vi "Set Serial Settings.vi"(8 "error in (no error)":errorcluster, 11 "LightBox in":refnum<class "LightBox.lvclass">=refnum) -> (0 "error out":errorcluster, 3 "LightBox out":refnum<class "LightBox.lvclass">)   [LabVIEW 2016, in "LightBox.lvclass"]
uses:
  LightBox.lvclass
  Quartz/Quartz.lvclass
  Desktop/platinum-modbus-driver/omega_engineering-platinum-modbus-driver-671bd10261c3/Labview Source Code/Platinum Serial Modbus/Platinum_MB_serMode.ctl
  Desktop/platinum-modbus-driver/omega_engineering-platinum-modbus-driver-671bd10261c3/Labview Source Code/Platinum Serial Modbus/Platinum_MB_serFlowControl.ctl
  Desktop/platinum-modbus-driver/omega_engineering-platinum-modbus-driver-671bd10261c3/Labview Source Code/Platinum Serial Modbus/Platinum_MB_SerHandle.ctl
  Desktop/platinum-modbus-driver/omega_engineering-platinum-modbus-driver-671bd10261c3/Labview Source Code/Platinum Serial Modbus/Platinum_MB_serParity.ctl
  LightBox.lvclass/LightBox.ctl
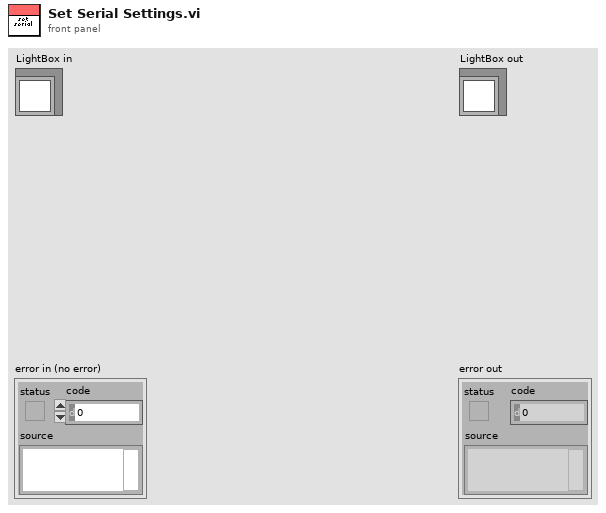
[diagram p1: front panel]
types:
  T1 = typedef "Platinum_MB_serFlowControl.ctl" = enum16{"None", "XON_XOFF", "RTS_CTS", "XON_XOFF_and_RTS_CTS", "DTR_DSR", "XON_XOFF_and_DTR_DSR"}
  T2 = typedef "Platinum_MB_serMode.ctl" = enum16{"RTU", "ASCII"}
  T3 = typedef "Platinum_MB_serParity.ctl" = enum16{"None", "Odd", "Even", "Mark", "Space"}
  T4 = typedef "Platinum_MB_SerHandle.ctl" = cluster{"VISAResourceName":string, "Mode":T2, "Timeout":u32, "FlowControl":T1, "Parity":T3, "BaudRate":u32, "SlaveAddress":u8}
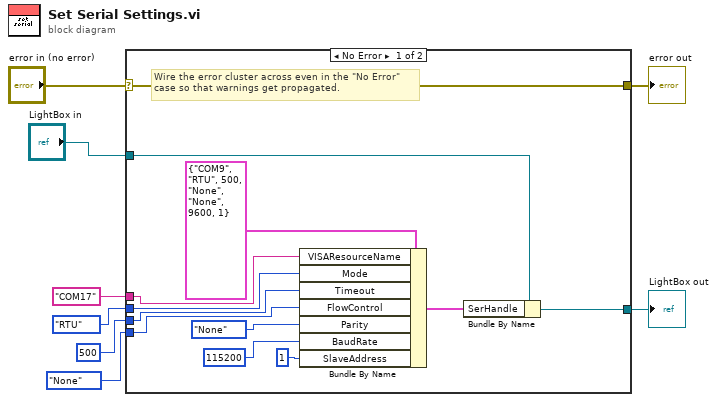
[diagram p0: block diagram]
diagram:
  n1 = case shown="No Error" "error in (no error)" {
    selector: "error in (no error)" -> [w20 w22]
    tunnel: [w20 w22] -> w7
    tunnel: [w18 w21] -> w5
    tunnel: "LightBox in" -> [w19 w21]
    tunnel: "COM17" ("VISAResourceName") -> [w15 _]
    tunnel: Platinum_MB_serMode."RTU" ("Mode") -> [w13 _]
    tunnel: u32 500 ("Timeout") -> [w14 _]
    tunnel: Platinum_MB_serFlowControl."None" ("FlowControl") -> [w12 _]
    frame No Error {
      # "Wire the error cluster across even in the \"No Error\"\ncase so that warnings get propagated."
      n2 = Bundle By Name(cluster=T4 {"VISAResourceName"="COM9", "Mode"=enum."RTU", "Timeout"=500, "FlowControl"=enum."None", "Parity"=enum."None", "BaudRate"=9600, "SlaveAddress"=1} ("SerHandle"), "VISAResourceName"=w15, "Mode"=w13, "Timeout"=w14, "FlowControl"=w12, "Parity"=Platinum_MB_serParity."None", "BaudRate"=u32 115200, "SlaveAddress"=u8 1) -> (w16:T4)
      n3 = Bundle By Name(cluster=w19, "SerHandle"=w16) -> (w18:refnum<class "LightBox.lvclass">)
    }
    frame Error {
    }
  }
  "error out" <- w7
  "LightBox out" <- w5
